vi "newFinalSingle.vi"(8 "error in (no error)":errorcluster, 11 "MagSpecCamera in":refnum<class "MagSpecCamera.lvclass">) -> (0 "error out":errorcluster, 3 "MagSpecCamera in":refnum<class "MagSpecCamera.lvclass">)   [LabVIEW 2013, in "MagSpecCamera.lvclass"]
uses:
  MagSpecCamera.lvclass
  MagSpecCamera.lvclass/MagSpecCamera.ctl
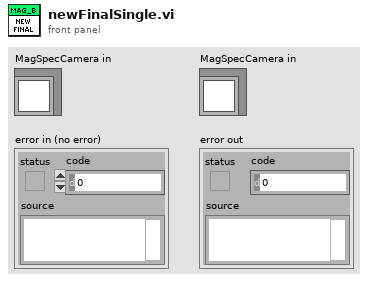
[diagram p1: front panel]
types:
  T1 = typedef "finalCalib--Cluster.ctl" = cluster{"X":dbl[][], "xi":dbl[][], "delta momentum":dbl, "Y":dbl[][], "yi":dbl[][], "angle (Y)":dbl[], "delta angle":dbl, "scale delta angle":dbl, "intraX":dbl, "intraY":dbl, "mask":dbl[][]}
  T2 = typedef "Calibration_Pixel_based.ctl" = cluster{"y1(pixel)":dbl[], "y2(pixel)":dbl[], "dp/B [MeV/C/B] (pixel)":dbl[], "energyDependence Input(pixel)":dbl[], "bending angle [deg](pixel)":dbl[], "total path(pixel)":dbl[], "pixel angle (y)(pixel)":dbl[], "energy dependence (pixel)":dbl[], "charge compensation (pixel)":dbl[], "Momentum [MeV/C](pixel)":dbl[], "angular compensation(pixel)":dbl[]}
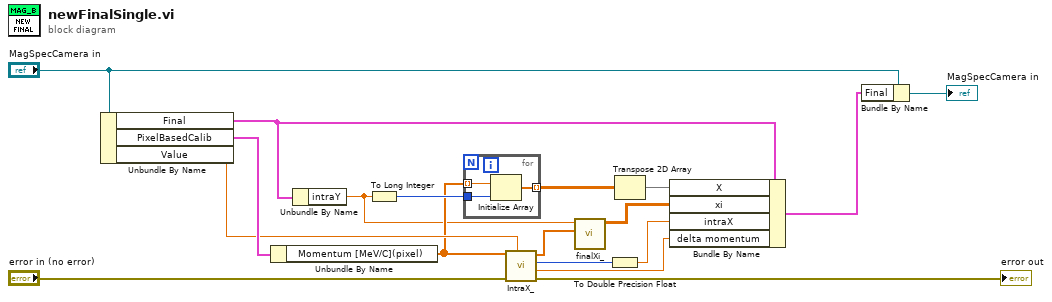
[diagram p0: block diagram]
diagram:
  n1 = Unbundle By Name("MagSpecCamera in") -> ("Final"=w15:T1, "PixelBasedCalib"=w12:T2, "Value"=w11:dbl)
  n2 = Unbundle By Name(w12) -> ("Momentum [MeV/C](pixel)"=w5:dbl[])
  n3 = Unbundle By Name(w15) -> ("intraY"=w3:dbl)
  n4 = To Long Integer(number=w3) -> (32bit integer=w8:i32)
  n5 = for {
    tunnel: w5 -> [w21] mode=indexing
    tunnel: w8 -> [w20]
    tunnel: [w19] -> w7 mode=indexing
    n6 = Initialize Array(w21, w20) -> (w19:dbl[])
  }
  n7 = call "IntraX_.vi"("DeltaE"=w11, "error in (no error)"="error in (no error)", "Momentum [MeV/C](pixel)"=w5) -> ("error out"=→"error out":errorcluster, "delta momentum"=w4:dbl, "IntraX"=w2:i32, "Ramp Pattern"=w9:dbl[])  [unwired: 5 in]
  n8 = call "finalXi_.vi"("Ramp Pattern"=w9, "intraY"=w3) -> ("Array"=w10:dbl[][])  [unwired: 9 in]
  n9 = To Double Precision Float(number=w2) -> (double precision float=w1:dbl)
  n10 = Transpose 2D Array(2D array=w7) -> (transposed array=w6:dbl[][])
  n11 = Bundle By Name(cluster=w15, "X"=w6, "xi"=w10, "intraX"=w1, "delta momentum"=w4) -> (w17:T1)
  n12 = Bundle By Name(cluster="MagSpecCamera in", "Final"=w17) -> (→"MagSpecCamera in":refnum<class "MagSpecCamera.lvclass">)
